vi "RT Error HandlerSam.vi"(8 "Ignore Errors":i32[](array[numeric]), 9 "Critical Errors":i32[](array[numeric]), 10 "error to process":errorcluster, 11 "queue in":refnum<queue>) -> (3 "queue out":refnum<queue>)   [LabVIEW 2014]
uses:
  controls/UI Data.ctl
  controls/RT Error MessageSam.ctl
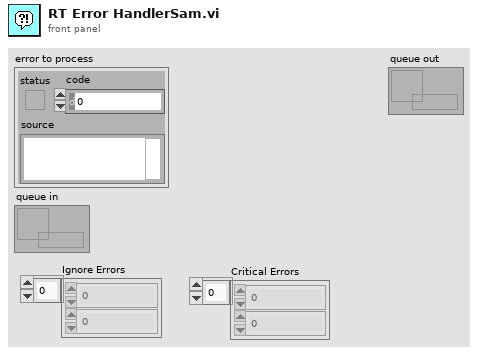
[diagram p1: front panel]
types:
  T1 = typedef "RT Error MessageSam.ctl" = enum16{"RT Non-Critical Error", "RT Critical Error"}
  T2 = typedef "UI Data.ctl" = cluster{"Message":string, "Data":variant}
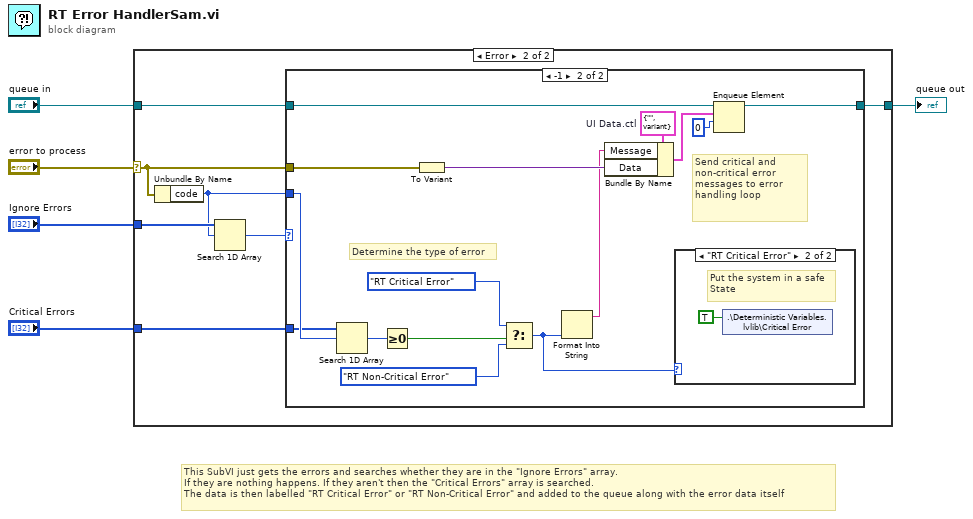
[diagram p0: block diagram]
diagram:
  # "This SubVI just gets the errors and searches whether they are in the \"Ignore Errors\" array. \nIf they are nothing happens. If they aren't then the \"Critical Errors\" array is searched.\nThe data is then labelled \"RT Critical Error\" or \"RT Non-Critical Error\" and added to the queue along with the error data itself"
  n1 = case shown="Error" "error to process" {
    selector: "error to process" -> [_ w8]
    tunnel: "Ignore Errors" -> [_ w13]
    tunnel: "Critical Errors" -> [_ w10]
    tunnel: "queue in" -> [w6 w9]
    tunnel: [w6 w7] -> w2
    frame No Error {
    }
    frame Error {
      n2 = Unbundle By Name(w8) -> ("code"=w11:i32)
      n3 = Search 1D Array(1D array=w13, element=w11) -> (index of element=w12:i32)  [unwired: 1 in]
      n4 = case shown="-1" w12 {
        tunnel: w11 -> [_ w29]
        tunnel: w10 -> [_ w26]
        tunnel: w9 -> [w14 w25]
        tunnel: w8 -> [_ w24]
        tunnel: [w14 w19] -> w7
        frame Default {
          # "Do nothing if error is categorized as \"Ignore Error\""
        }
        frame -1 {
          w21 = T2 {"Message"="", "Data"=variant}  # UI Data.ctl
          # "Send critical and non-critical error messages to error handling loop"
          # "Determine the type of error"
          n5 = Search 1D Array(1D array=w26, element=w29) -> (index of element=w28:i32)  [unwired: 1 in]
          n6 = Greater Or Equal To 0?(x=w28) -> (x >= 0?=w27:bool)
          n7 = To Variant(anything=w24) -> (Variant=w23:variant)
          n8 = Select(t=RT_Error_MessageSam."RT Critical Error", s=w27, f=RT_Error_MessageSam."RT Non-Critical Error") -> (s? t:f=w15:T1)
          n9 = Format Into String "Format Into String"(w15) -> (resulting string=w22:string)  [unwired: 3 in, 1 out]
          n10 = Bundle By Name(cluster=w21, "Message"=w22, "Data"=w23) -> (w20:T2)
          n11 = case shown="\"RT Critical Error\"" w15 {
            frame "RT Non-Critical Error", Default {
            }
            frame "RT Critical Error" {
              # "Put the system in a safe\nState"
              n12 = shared-variable ".\\Deterministic Variables.lvlib\\Critical Error"(TRUE ("Critical Error")) -> ()  [unwired: 1 in, 1 out]
            }
          }
          n13 = Enqueue Element(queue=w25, element=w20, timeout in ms (-1)=0) -> (queue out=w19:refnum<queue>)  [unwired: 1 in, 2 out]
        }
      }
    }
  }
  "queue out" <- w2
